vi "PiezoJena-pos-Command.vi"(11 "NanoBox pos":dbl(slide) scale=0.0..120.0) -> (3 "SIAMScript":T2(array[cluster]) {"command" format="%x" items=["read_x-Motor_status_ticket"=17305600, "init_x-Motor"=17760263, "read_x-Motor_absolute_ticket"=16781312, "move_x-Motor_absolute"=16777217, "move_x-Motor_relative"=16842753, "read_x-Motor_speed"=16977920, "set_x-Motor_speed"=16973825, "read_y-Motor_status_ticket"=18354176, "init_y-Motor"=18808839, "read_y-Motor_absolute_ticket"=17829888, "move_y-Motor_absolute"=17825793, "move_y-Motor_relative"=17891329, "read_y-Motor_speed"=18026496, "set_y-Motor_speed"=18022401, "read_z-Motor_status_ticket"=19402752, "init_z-Motor"=19857415, "stop_z-Motor"=19857423, "start_z-Motor"=19857422, "read_z-Motor_absolute_ticket"=18878464, "move_z-Motor_absolute"=18874369, "move_z-Motor_relative"=18939905, "read_Objective_status_ticket"=20451328, "init_Objective"=20905991, "read_Objective_absolute_ticket"=19927040, "move_Objective_absolute"=19922945, "move_Objective_relative"=19988481, "read_Objective-Motor_speed"=20123648, "set_Objective-Motor_speed"=20119553, "read_Filter_status_ticket"=21499904, "init_Filter"=21954567, "read_Filter_absolute_ticket"=20975616, "move_Filter_absolute"=20971521, "move_Filter_relative"=21037057, "read_Filter-Motor_speed"=21172224, "set_Filter-Motor_speed"=21168129, "read_Trans-Rad_status_ticket"=22548480, "init_Trans-Rad"=23003143, "read_Trans-Rad_absolute_ticket"=22024192, "move_Trans-Rad_absolute"=22020097, "move_Trans-Rad_relative"=22085633, "read_Trans-Motor_speed"=22220800, "set_Trans-Motor_speed"=22216705, "read_FRET_status_ticket"=23597056, "init_FRET"=24051719, "read_FRET_absolute_ticket"=23072768, "move_FRET_absolute"=23068673, "move_FRET_relative"=23134209, "read_FRET-Motor_speed"=23269376, "set_FRET-Motor_speed"=23265281, "read_SI-Rad_status_ticket"=24645632, "init_SI-Rad"=25100295, "read_SI-Rad_absolute_ticket"=24121344, "move_SI-Rad_absolute"=24117249, "move_SI-Rad_relative"=24182785, "read_SI-Rad_speed"=24317952, "set_SI-Rad_speed"=24313857, "I2C-write"=335544321, "I2C-read"=335548416, "UART0-VC-Baud-write"=469958657, "UART0-VC-Baud-read"=469962752, "UART0-VC-write"=469762049, "UART0-VC-write-Var"=469762051, "UART0-VC-read"=469766144, "UART0-VC-read-Var"=469766146, "UART1-TSM-write"=486539265, "UART1-TSM-read"=486543360, "UART2-write"=503316481, "UART2-read"=503320576, "UART3-write"=520093697, "UART3-read"=520097792, "end_no_ticket"=4027514895, "end_ticket"=4027518991, "IO-read_bank0"=3489665024, "IO-write_bank0"=3489660929, "IO-read_bank1"=3506442240, "IO-write_bank1"=3506438145, "DA0-0_LED365"=2684354561, "DA0-1_LED385"=2685403137, "DA0-2_LED440"=2686451713, "DA0-3_LED470"=2687500289, "DA0-4_LED510"=2688548865, "DA0-5_LED550"=2689597441, "DA0-6_LED590"=2690646017, "DA0-7_LED640"=2691694593, "DA1-0_LED-R"=2701131777, "DA1-1_LED-G"=2702180353, "DA1-2_LED-B"=2703228929, "DA1-3_LED-AF"=2704277505, "DA1-4"=2705326081, "DA1-5"=2706374657, "DA1-6"=2707423233, "DA1-7"=2708471809, "DA2-Laser0"=2717908993, "DA2-Laser1"=2718957569, "DA2-Laser2"=2720006145, "DA2-Laser3"=2721054721, "DA2-Laser4"=2722103297, "Analog-read_AD0-0"=2818576384, "Analog-read-store_AD0-0"=2818572290, "IO-delay_bank0"=3489923073, "IO-delay_bank0_fromVar"=3489923075, "read_cam_clock"=3289124864, "store_cam_clock"=3289120770, "read_cam_phase"=3289190400, "store_cam_phase"=3289190402, "Read ticks"=4027518976, "Read ticks to var"=4027518978, "Read IP"=4043313152, "Read IP into var"=4043313154, "Set IP from var"=4043309059, "Set IP from var, relative"=4043313155, "decrement_branchRel_if_equal"=4043374945, "decrement_branchRel_if_greaterequal"=4043375201, "decrement_branchRel_if_greaterequal_withTicket"=4043379297, "decrement_branchRel_if_smaller"=4043375457, "increment_branchRel_if_smaller"=4043375473, "readVar"=4060090368, "writeVar"=4060086273, "readVar_and_copy_to_var2"=4060086275, "loadVar2_andcopy_var1"=4060086276, "math_addToVariable"=4076863488, "math_addVToVariable"=4076863489, "math_subToVariable"=4076863490, "math_subVToVariable"=4076863491, "math_multToVariable"=4076863492, "math_multvToVariable"=4076863493, "math_divideToVariable"=4076863494, "math_divideVToVariable"=4076863495, "math_modToVariable"=4076863496, "math_modVToVariable"=4076863497, "logic_and"=4093640704, "logic_or"=4093640706, "logic_xor"=4093640708, "bitshift"=4093640712, "set_1Galvo"=101712113, "set_x-Galvo"=102760689, "set_y-Galvo"=103809265, "set_z-Fokus"=104857841, "set_1Galvo_position-only"=101711937, "set_x-Galvo_position-only"=102760513, "set_y-Galvo_position-only"=103809089, "set_z-Fokus_position-only"=104857665, "set_x-Galvo_position-only_ticket"=102764609, "set_y-Galvo_position-only_ticket"=103813185, "set_z-Fokus_position-only_ticket"=104861761, "set_x-Galvo_relativ-only"=102760577, "set_y-Galvo_relativ-only"=103809153, "set_z-Fokus_relativ-only"=104857729, "set_x-Galvo_speed-only"=102760481, "set_y-Galvo_speed-only"=103809057, "set_z-Fokus_speed-only"=104857633, "read_1Galvo_ticket"=101716032, "read_x-Galvo_ticket"=102764608, "read_y-Galvo_ticket"=103813184, "read_z-Focus_ticket"=104861760, "x-Galvo_pos_fromVar"=102760515, "y-Galvo_pos_fromVar"=103809091, "z-Focus_pos_fromVar"=104857667, "Servo0"=67108865, "Servo0-enable"=68091911, "Servo0-disable"=68091919, "Servo1"=68157441, "Servo1-enable"=69140487, "Servo1-disable"=69140495, "xCounter-Enable"=202309639, "xCounter-Bits"=201523201, "xCounter-Read"=201330688]; "P4" format="%x"; "P3" format="%x"; "P2" format="%x"; "P1" format="%x"})   [LabVIEW 2011]
uses:
  Program Files/SIAM_test_Standalone/SIAM/SIAM_command.ctl
panel:
  out "unsigned byte array":u8[](array[numeric]) format="%x"
  out "*(type *) &x":u32[](array[numeric]) format="%.0x"
  out "resulting string":string
  # "0D0A0000"
  # "706F732C"
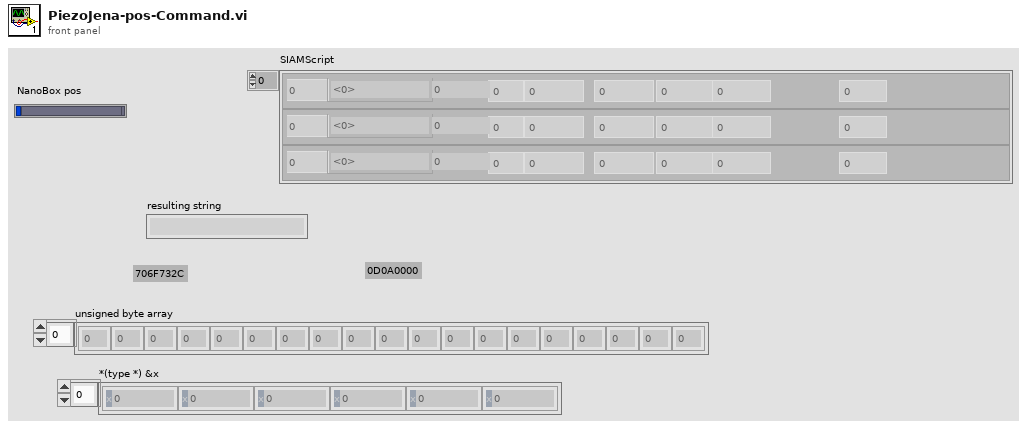
[diagram p1: front panel]
types:
  T1 = typedef "SIAM_command.ctl" = u32
  T2 = cluster{"Delay 10µs":u32, "command":T1, "P0":i32, "P1":i32, "P2":i32, "P3":i32, "P4":i32, "P5-ticket":i32}[]
  T3 = cluster{"Delay 10µs":u32, "command":T1, "P0":i32, "P1":i32, "P2":i32, "P3":i32, "P4":i32, "P5-ticket":i32}
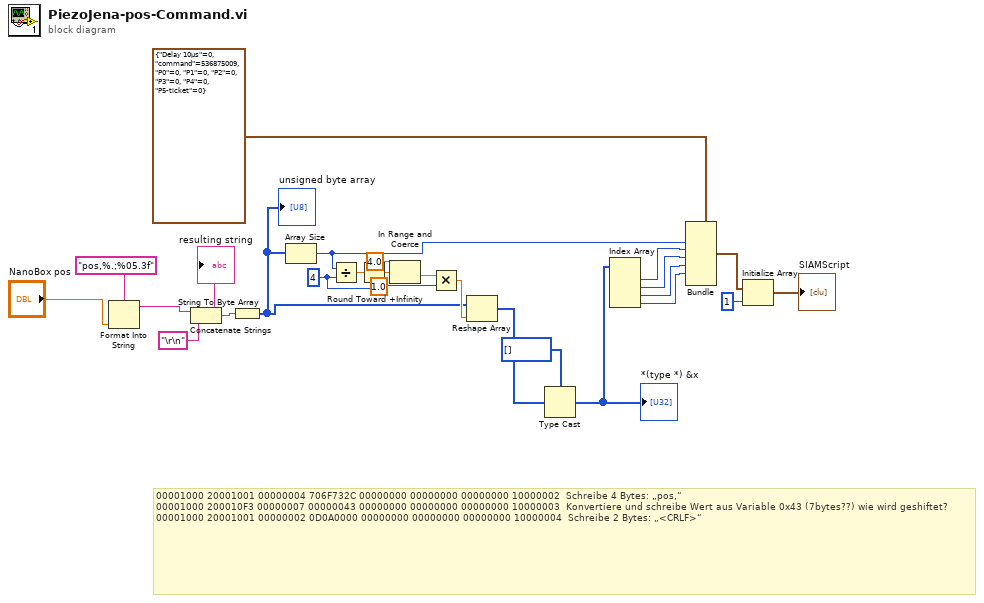
[diagram p0: block diagram]
diagram:
  w15 = 4 ("y")
  # "00001000 20001001 00000004 706F732C 00000000 00000000 00000000 10000002  Schreibe 4 Bytes: „pos,“\n00001000 200010F3 00000007 00000043 00000000 00000000 00000000 10000003  Konvertiere und schreibe Wert aus Variable 0x43 (7bytes??) wie wird geshiftet?\n00001000 20001001 00000002 0D0A0000 00000000 00000000 00000000 10000004  Schreibe 2 Bytes: „<CRLF>“"
  n1 = Format Into String(format string="pos,%.;%05.3f", "NanoBox pos") -> (resulting string=w21:string)  [unwired: 2 in, 1 out]
  n2 = Concatenate Strings(w21, "\r\n") -> (w19:string)
  "resulting string" <- w19
  n3 = String To Byte Array(string=w19) -> (unsigned byte array=w13:u8[])
  "unsigned byte array" <- w13
  n4 = Array Size(array=w13) -> (size(s)=w18:i32)
  n5 = Divide(x=w18, y=w15) -> (x/y=w17:dbl)
  n6 = Round Toward +Infinity(x=w17) -> (ceil(x): smallest int >= x=w16:dbl)
  n7 = In Range and Coerce(upper limit=4.0, x=w16, lower limit=1.0) -> (coerced(x)=w11:dbl)  [unwired: 1 out]
  n8 = Multiply(x=w11, y=w15) -> (x*y=w14:dbl)
  n9 = Reshape Array(w13, w14) -> (w12:u8[])
  n10 = Type Cast(type=u32[] [], x=w12) -> (*(type *) &x=w8:u32[])
  "*(type *) &x" <- w8
  n11 = Index Array(array=w8) -> (element #1=w7:u32, element #2=w6:u32, element #3=w5:u32, element #4=w4:u32)  [unwired: 4 in]
  n12 = Bundle(cluster=T3 {"Delay 10µs"=0, "command"=536875009, "P0"=0, "P1"=0, "P2"=0, "P3"=0, "P4"=0, "P5-ticket"=0} ("Cluster"), "P0"=w18, "P1"=w7, "P2"=w6, "P3"=w5, "P4"=w4) -> (w3:T3)  [unwired: 3 in]
  n13 = Initialize Array(w3, 1 ("dimension size")) -> (→"SIAMScript":T2)
